vi "count types.vi"() -> (3 "type count":i32)   [LabVIEW 2013, in "tag bus.lvlib" / "tag descriptor.lvclass"]
doc: "Indicates the number of types supported by the framework."
uses:
  tag descriptor.lvclass
  Data Type.ctl
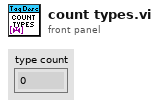
[diagram p1: front panel]
types:
  T1 = typedef "tag bus.lvlib/tag descriptor.lvclass/Data Type.ctl" = enum16{"Double", "Single", "I64", "I32", "I16", "I8", "U64", "U32", "U16", "U8", "Boolean", "String", "Array of Double", "Array of Single", "Array of I64", "Array of I32", "Array of I16", "Array of I8", "Array of U64", "Array of U32", "Array of U16", "Array of U8", "Array of Boolean", "Array of String"}
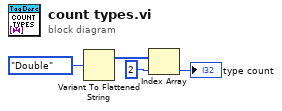
[diagram p0: block diagram]
diagram:
  n1 = Variant To Flattened String(Variant=Data_Type."Double" ("Data Type")) -> (1:w4:i16[])  [unwired: 1 out]
  n2 = Index Array(array=w4, index=2) -> (element=→"type count":i16)
